vi "open.vi"(1 "ItemNames in":string[][](array[string])) -> (0 "ItemNames out":string[][](array[string]))   [LabVIEW 2019]
uses:
  <vilib>/Utility/file.llb/Read Delimited Spreadsheet (string).vi
panel:
  out "Array 2":string[][](array[string])
  out "error out":errorcluster
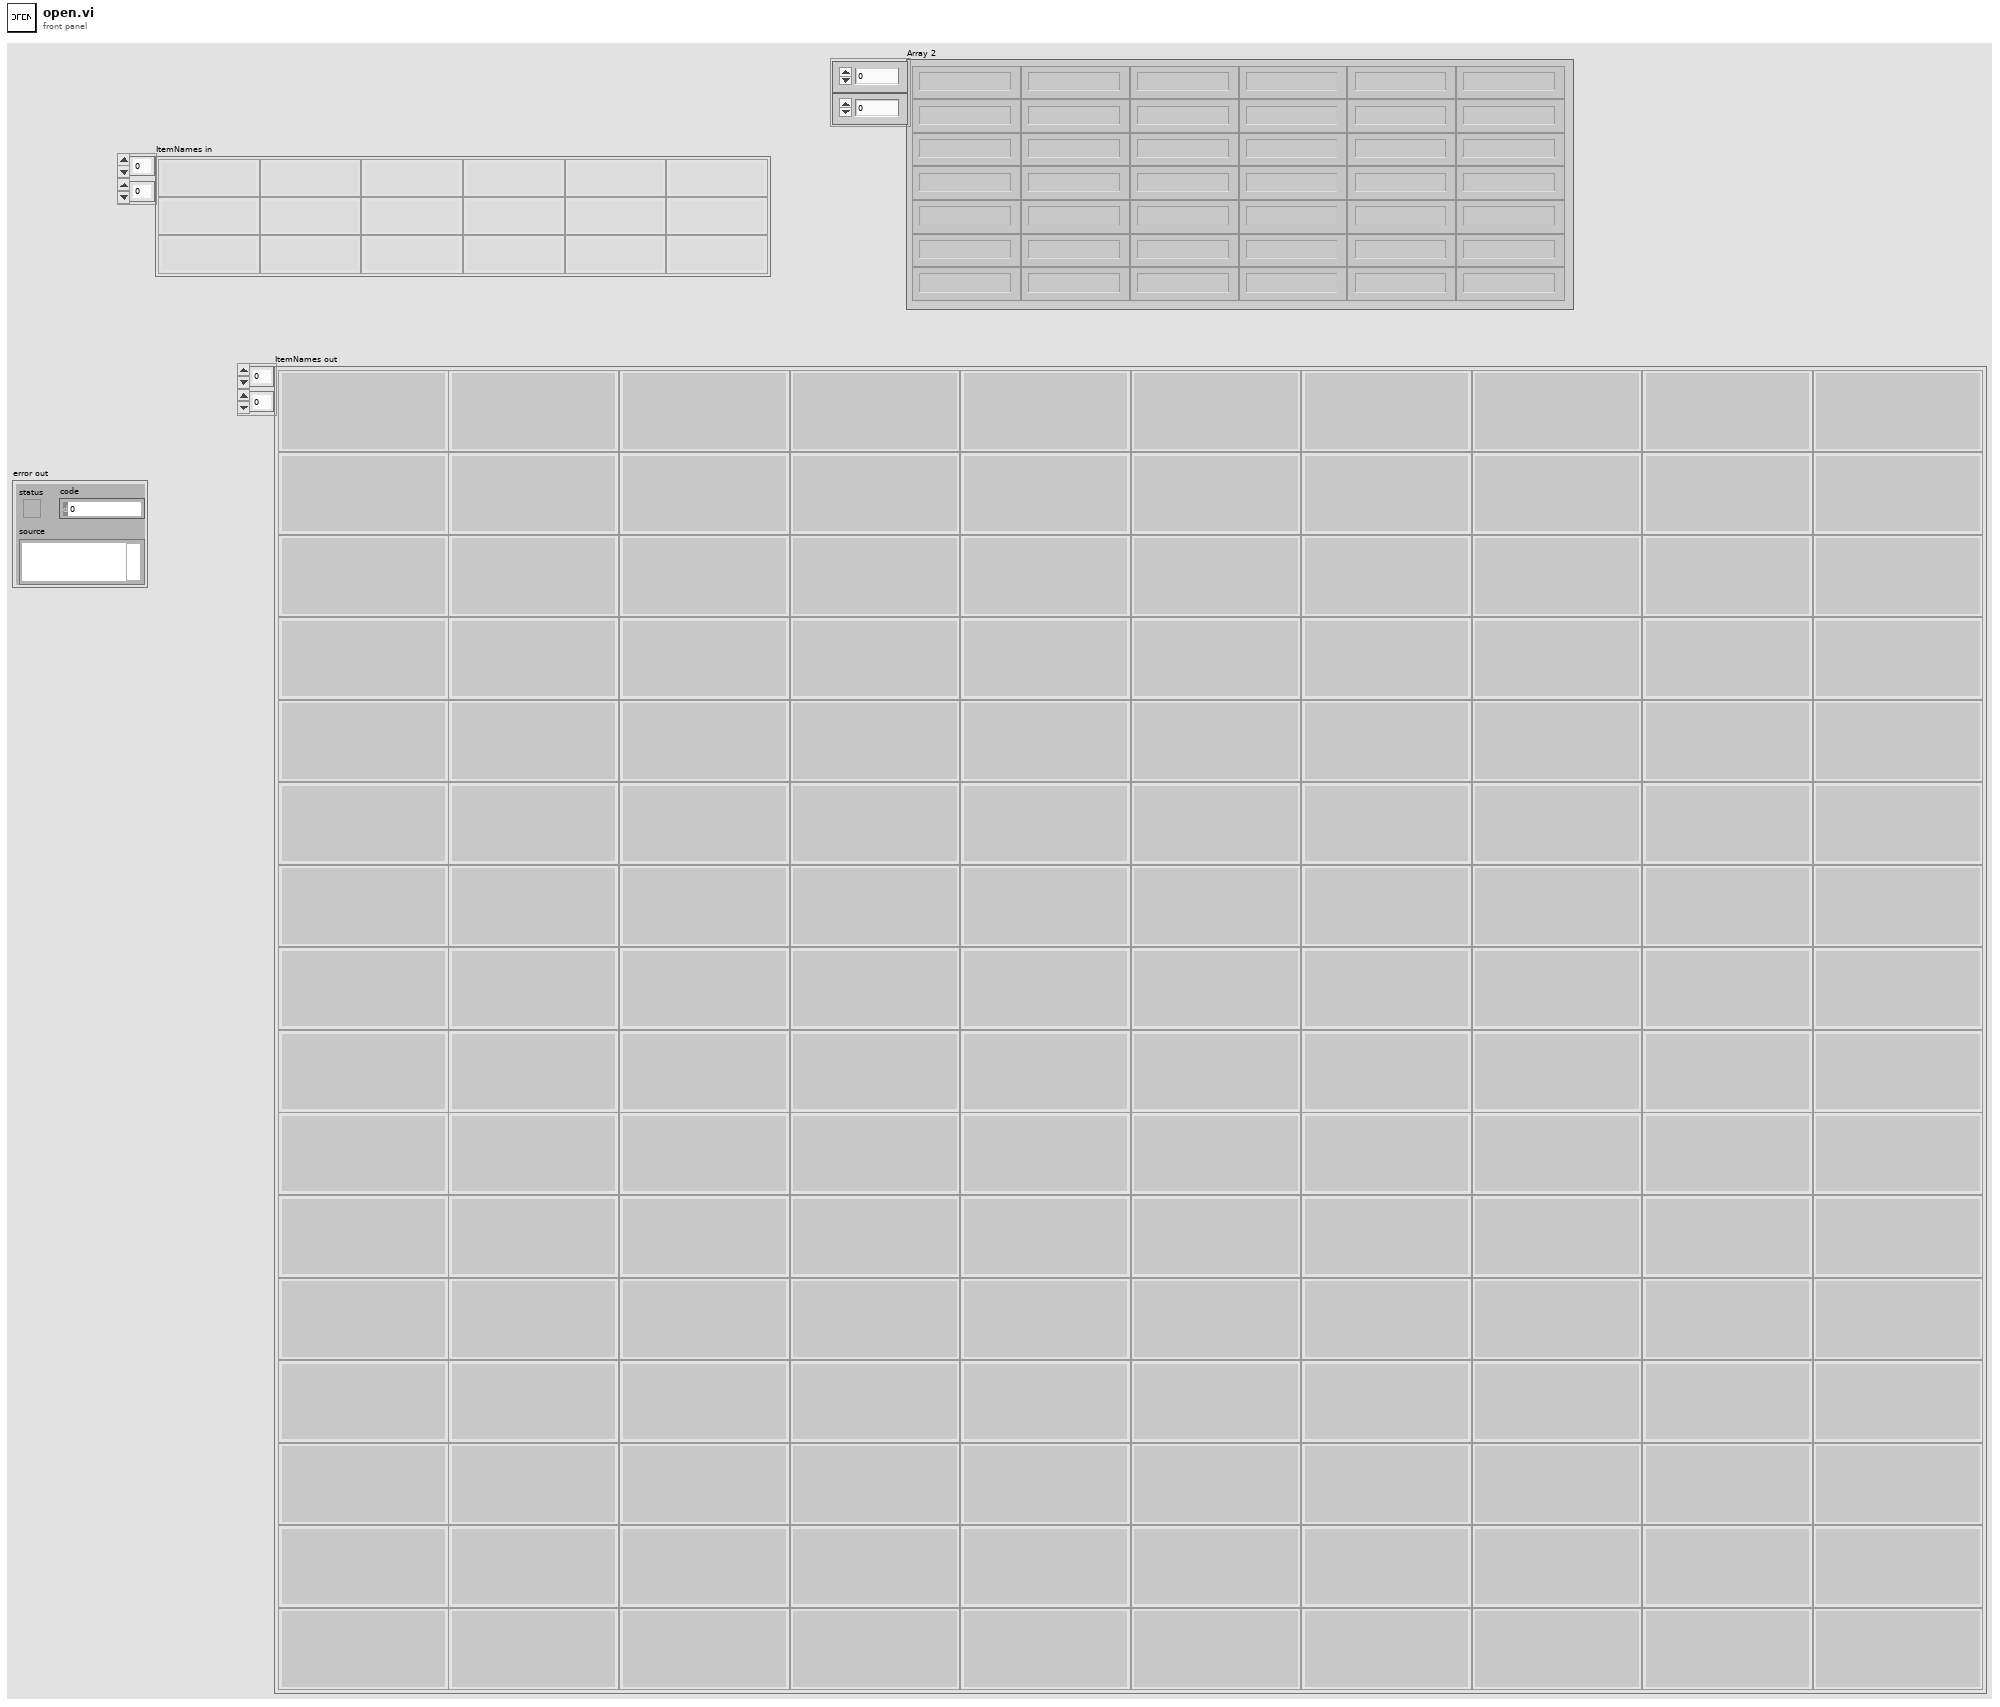
[diagram p1: front panel]
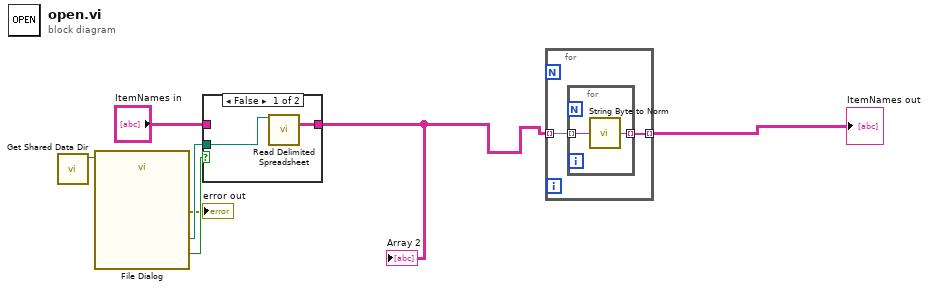
[diagram p0: block diagram]
diagram:
  n1 = call "Get Shared Data Dir.vi"() -> ("Data Directory Path"=w4:path)  [unwired: 2 in, 1 out]
  n2 = call "File Dialog"("start path"=w4) -> ("selected path"=w6:path, "cancelled"=w7:bool, "error out"=→"error out":errorcluster)  [unwired: 11 in, 1 out]
  n3 = case shown="False" w7 {
    tunnel: w6 -> [w9 _]
    tunnel: [w8 w10] -> w1
    tunnel: "ItemNames in" -> [_ w10]
    frame False {
      n4 = call-poly <vilib>:"Read Delimited Spreadsheet.vi"("file path (dialog if empty)"=w9) -> ("all rows"=w8:string[][])  [unwired: 9 in, 5 out]
    }
    frame True {
    }
  }
  "Array 2" <- w1
  n5 = for {
    tunnel: w1 -> [w12] mode=indexing
    tunnel: [w11] -> w2 mode=indexing
    n6 = for {
      tunnel: w12 -> [w14] mode=indexing
      tunnel: [w13] -> w11 mode=indexing
      n7 = call "String Byte to Norm.vi"("Byte String In"=w14) -> ("String Out"=w13:string)
    }
  }
  "ItemNames out" <- w2
